vi "RestrictString.vi"(9 "NumberOfString":i32=5, 10 "StringIn":string, 11 "NewString":string) -> (2 "StringOut":string)   [LabVIEW 2015]
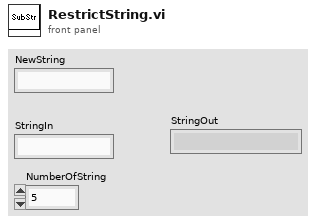
[diagram p1: front panel]
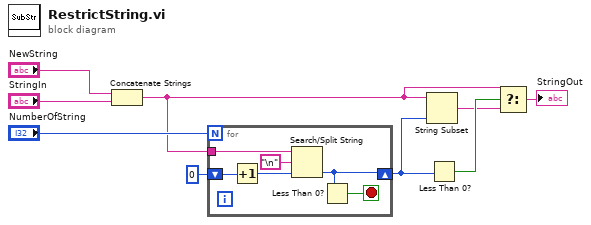
[diagram p0: block diagram]
diagram:
  n1 = Concatenate Strings("NewString", "StringIn") -> (w3:string)
  n2 = for {
    N: "NumberOfString" -> [_]
    tunnel: w3 -> [w15]
    shift-right: [w10] -> w5
    shift-left: 0 ("offset of match") -> [w12]
    stop <- w13 stop-if-true
    n3 = Increment(x=w12) -> (x+1=w11:i32)
    n4 = Search/Split String(string=w15, search string/char (-)="\n", offset (0)=w11) -> (offset of match=w10:i32)  [unwired: 2 out]
    n5 = Less Than 0?(x=w10) -> (x < 0?=w13:bool)
  }
  n6 = String Subset(string=w3, length (rest)=w5) -> (substring=w2:string)  [unwired: 1 in]
  n7 = Less Than 0?(x=w5) -> (x < 0?=w4:bool)
  n8 = Select(t=w3, s=w4, f=w2) -> (s? t:f=→"StringOut":string)
